vi "Check for Log Folder (No Objects).vi"() -> ()   [LabVIEW 2012]
uses:
  Global/File Locations.vi
panel:
  out "error out 2":errorcluster
  out "error out":errorcluster
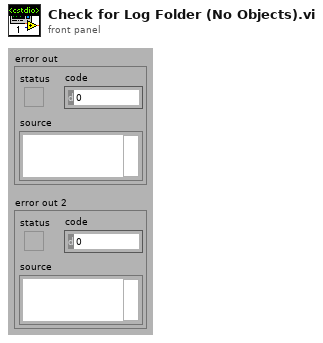
[diagram p1: front panel]
types:
  T1 = enum16{"open", "replace", "create", "open or create", "replace or create", "replace or create with confirmation"}
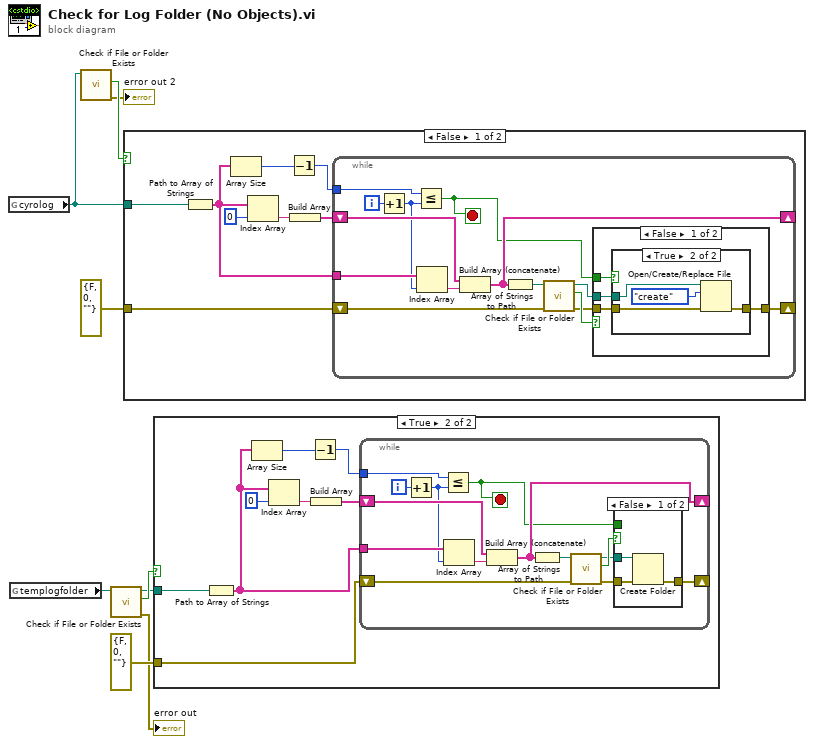
[diagram p0: block diagram]
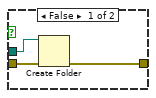
[diagram p2: hidden frame]
diagram:
  n1 = global read "File Locations.vi" "cyrolog"() -> (w2:path)
  n2 = global read "File Locations.vi" "templogfolder"() -> (w9:path)
  n3 = call <vilib>:"Check if File or Folder Exists.vi"("path"=w2) -> ("error out"=→"error out 2":errorcluster, "file or folder exists?"=w7:bool)  [unwired: 1 in, 8 out]
  n4 = call <vilib>:"Check if File or Folder Exists.vi"("path"=w9) -> ("error out"=→"error out":errorcluster, "file or folder exists?"=w8:bool, "dup path"=w4:path)  [unwired: 1 in, 7 out]
  n5 = case shown="False" w7 {
    tunnel: w2 -> [w17 _]
    tunnel: errorcluster {"status"=FALSE, "code"=0, "source"=""} ("error out") -> [w10 _]
    frame False {
      n6 = Path to Array of Strings(0:w17) -> (2:w14:string[])  [unwired: 1 out]
      n7 = Array Size(array=w14) -> (size(s)=w16:i32)
      n8 = Index Array(array=w14, index=0) -> (element=w11:string)
      n9 = Decrement(x=w16) -> (x-1=w15:i32)
      n10 = Build Array(w11) -> (w12:string[])
      n11 = while {
        tunnel: w14 -> [w29]
        tunnel: w15 -> [w25]
        shift-right: [w27] -> _
        shift-left: w12 -> [w31]
        shift-right: [w18] -> _
        shift-left: w10 -> [w20]
        i -> [w30]
        stop <- w21 stop-if-true
        n12 = Increment(x=w30) -> (x+1=w24:i32)
        n13 = Less Or Equal?(x=w25, y=w24) -> (x <= y?=w21:bool)
        n14 = Index Array(array=w29, index=w24) -> (element=w28:string)
        n15 = Build Array (concatenate)(w31, w28) -> (w27:string[])
        n16 = Array of Strings to Path(0:w27) -> (2:w26:path)  [unwired: 1 out]
        n17 = call <vilib>:"Check if File or Folder Exists.vi"("error in (no error)"=w20, "path"=w26) -> ("error out"=w19:errorcluster, "file or folder exists?"=w23:bool, "dup path"=w22:path)  [unwired: 7 out]
        n18 = case shown="False" w23 {
          tunnel: w22 -> [w35 _]
          tunnel: w21 -> [w34 _]
          tunnel: w19 -> [w33 w43]
          tunnel: [w32 w43] -> w18
          frame False {
            n19 = case shown="True" w34 {
              tunnel: w35 -> [w38 w42]
              tunnel: w33 -> [w36 w41]
              tunnel: [w37 w40] -> w32
              frame False {
                n20 = Create Folder(path (use dialog)=w38, error in=w36) -> (error out=w37:errorcluster)  [unwired: 3 out]
              }
              frame True {
                n21 = Open/Create/Replace File(file path (use dialog)=w42, error in=w41, operation (0:open)=T1."create") -> (error out=w40:errorcluster)  [unwired: 5 out]
              }
            }
          }
          frame True {
          }
        }
      }
    }
    frame True {
    }
  }
  n22 = case shown="True" w8 {
    tunnel: errorcluster {"status"=FALSE, "code"=0, "source"=""} ("error out") -> [_ w45]
    tunnel: w4 -> [_ w44]
    frame False {
    }
    frame True {
      n23 = Path to Array of Strings(0:w44) -> (2:w49:string[])  [unwired: 1 out]
      n24 = Array Size(array=w49) -> (size(s)=w51:i32)
      n25 = Index Array(array=w49, index=0) -> (element=w46:string)
      n26 = Decrement(x=w51) -> (x-1=w50:i32)
      n27 = Build Array(w46) -> (w47:string[])
      n28 = while {
        tunnel: w49 -> [w63]
        tunnel: w50 -> [w59]
        shift-right: [w61] -> _
        shift-left: w47 -> [w65]
        shift-right: [w52] -> _
        shift-left: w45 -> [w54]
        i -> [w64]
        stop <- w55 stop-if-true
        n29 = Increment(x=w64) -> (x+1=w58:i32)
        n30 = Less Or Equal?(x=w59, y=w58) -> (x <= y?=w55:bool)
        n31 = Index Array(array=w63, index=w58) -> (element=w62:string)
        n32 = Build Array (concatenate)(w65, w62) -> (w61:string[])
        n33 = Array of Strings to Path(0:w61) -> (2:w60:path)  [unwired: 1 out]
        n34 = call <vilib>:"Check if File or Folder Exists.vi"("error in (no error)"=w54, "path"=w60) -> ("error out"=w53:errorcluster, "file or folder exists?"=w57:bool, "dup path"=w56:path)  [unwired: 7 out]
        n35 = case shown="False" w57 {
          tunnel: w56 -> [w68 _]
          tunnel: w55 -> [_ _]
          tunnel: w53 -> [w67 w69]
          tunnel: [w66 w69] -> w52
          frame False {
            n36 = Create Folder(path (use dialog)=w68, error in=w67) -> (error out=w66:errorcluster)  [unwired: 3 out]
          }
          frame True {
          }
        }
      }
    }
  }
